vi "Get Overload Protection State.vi"(8 "error in (no error)":errorcluster, 11 "VISA resource name":refnum<visa-resource-name>) -> (0 "error out":errorcluster, 2 "Detected State":dbl format="%.4f", 3 "VISA resource name out":refnum<visa-resource-name>)   [LabVIEW 2014, in "Fluke 5XXX Series Multicalibrators.lvlib"]
doc: "This VI returns the detected state of scope overload protection.\n\nNote:\n\nThis VI is available only for instrument models 5500A and 5520A with oscilloscope option SC600 (SC1100)."
uses:
  Fluke 5XXX Series Multicalibrators.lvlib
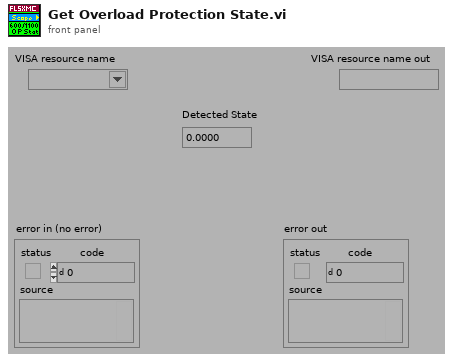
[diagram p1: front panel]
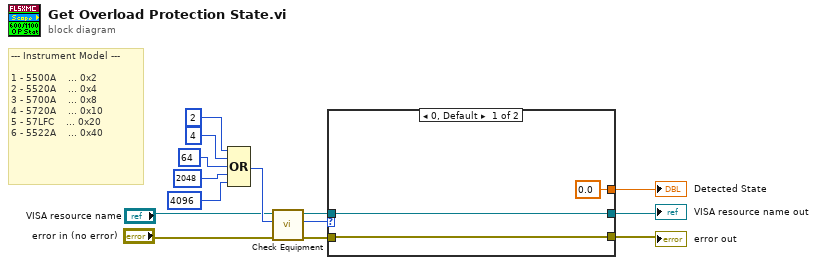
[diagram p0: block diagram]
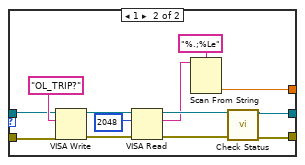
[diagram p2: hidden frame]
diagram:
  # "--- Instrument Model ---\n\n1 - 5500A    ... 0x2\n2 - 5520A    ... 0x4\n3 - 5700A    ... 0x8\n4 - 5720A    ... 0x10\n5 - 57LFC    ... 0x20\n6 - 5522A    ... 0x40"
  n1 = Compound Arithmetic op=OR(2 ("Numeric"), 4 ("Numeric"), 64 ("Numeric"), 2048 ("Numeric"), 4096 ("Numeric")) -> (w7:i32)
  n2 = call "Check Equipment.vi"("error in (no error)"="error in (no error)", "Bit Mask"=w7, "VISA resource name"="VISA resource name") -> ("error out"=w11:errorcluster, "Present?"=w10:u32, "VISA resource name out"=w9:refnum<visa-resource-name>)  [unwired: 6 in]
  n3 = case shown="0, Default" w10 {
    tunnel: [w16 w20] -> w3
    tunnel: w11 -> [w17 w22]
    tunnel: w9 -> [w16 w19]
    tunnel: [w17 w21] -> w4
    tunnel: [0.0 w18] -> w2
    frame 0, Default {
    }
    frame 1 {
      n4 = VISA Write(VISA resource name=w19, write buffer="OL_TRIP?", error in (no error)=w22) -> (VISA resource name out=w28:refnum<visa-resource-name>, error out=w27:errorcluster)  [unwired: 1 out]
      n5 = VISA Read(VISA resource name=w28, byte count=u32 2048 ("byte count (0)"), error in (no error)=w27) -> (VISA resource name out=w25:refnum<visa-resource-name>, read buffer=w24:string, error out=w26:errorcluster)  [unwired: 1 out]
      n6 = Scan From String(format string="%.;%Le", input string=w24) -> (output 1=w18:dbl)  [unwired: 3 in, 3 out]
      n7 = call "Check Status.vi"("VISA resource name"=w25, "error in (no error)"=w26) -> ("VISA resource name out"=w20:refnum<visa-resource-name>, "error out"=w21:errorcluster)  [unwired: 12 in]
    }
  }
  "Detected State" <- w2
  "VISA resource name out" <- w3
  "error out" <- w4
